vi "MGCC_Resync_main.vi"() -> ()   [LabVIEW 2016]
doc: "-----------------------------------------------------------------------------------------------------------------------\nCopyright <2019> <The University of Tennessee at Knoxville and the University of Tennessee Research Foundation>\nThis software is released under BSD-3 \nhttps://opensource.org/licenses/BSD-3-Clause \nAdditional license options available at https://utrf.tennessee.edu/industry/sample-agreements/\n-----------------------------------------------------------------------------------------------------------------------\n\nSimplified version of resynchronization, without support on dynamic boundary"
uses:
  Finite State Machine/Sub-VIs/MGCC_FntStaMach_gobal.vi
  <vilib>/Utility/error.llb/Error Cluster From Error Code.vi
  Communication/Global communication output.vi
  MGCC_Resync_global.vi
  Communication/Global communication.vi
  <vilib>/ErrorRing/Error Ring.xnode
panel:
  out "Resync Iterations":i16
  out "Critical_switch_first":i16
  out "resync_switch":i32[](array[numeric])
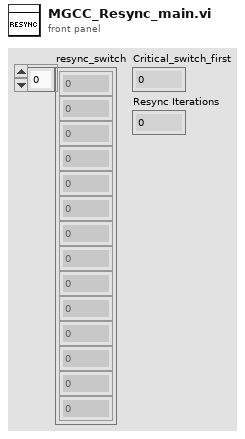
[diagram p1: front panel]
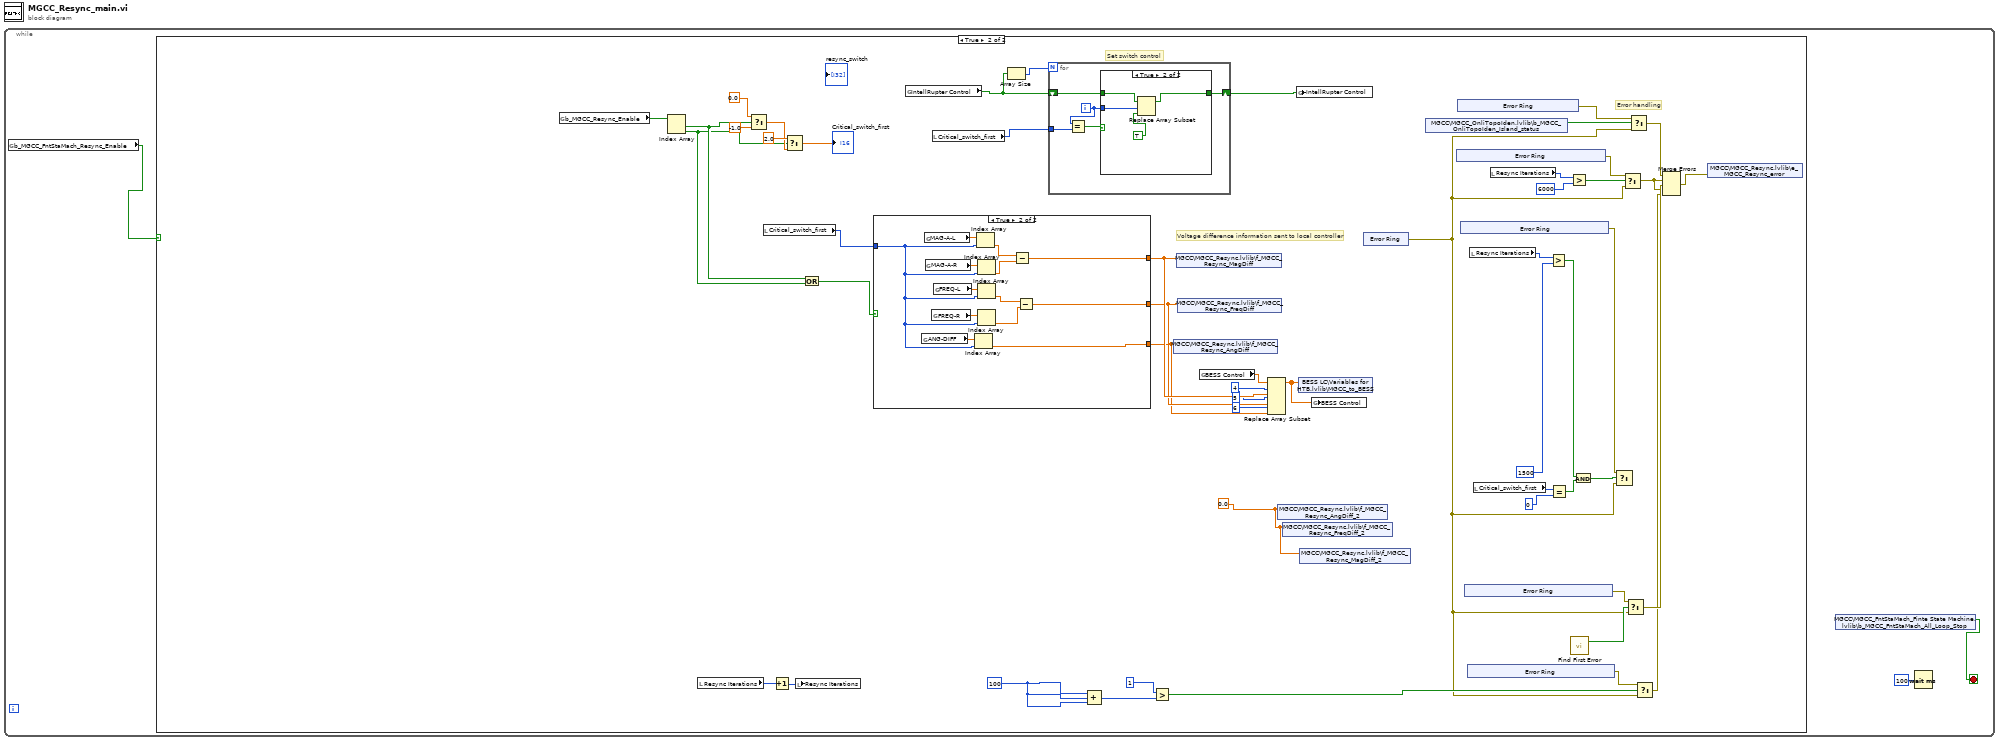
[diagram p0: block diagram]
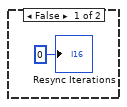
[diagram p2: hidden frame]
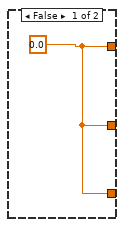
[diagram p3: hidden frame]
diagram:
  n1 = while {
    stop <- w2 stop-if-true
    n2 = global read "MGCC_FntStaMach_gobal.vi" "b_MGCC_FntStaMach_Resync_Enable"() -> (w1:bool)
    n3 = case shown="True" w1 {
      frame False {
        "Resync Iterations" <- i16 0 ("Resync Iterations")
      }
      frame True {
        w35 = 100 ("y")
        w28 = 0.0
        # "Set switch control"
        # "Error handling"
        # "Voltage difference information sent to local controller"
        n4 = global read "MGCC_Resync_global.vi" "b_MGCC_Resync_Enable"() -> (w18:bool[])
        n5 = Index Array(array=w18) -> (element #1=w9:bool, element #2=w8:bool)  [unwired: 2 in]
        n6 = local read "Resync Iterations"() -> (w56:i16)
        n7 = Select(t=0.0 ("f"), s=w9, f=-1.0) -> (s? t:f=w15:dbl)
        n8 = local read "Critical_switch_first"() -> (w12:i16)
        n9 = Increment(x=w56) -> (x+1=w55:i16)
        n10 = Select(t=2.0 ("f"), s=w8, f=w15) -> (s? t:f=→"Critical_switch_first":dbl)
        n11 = local write "Resync Iterations"(w55) -> ()
        n12 = Or(x=w9, y=w8) -> (x .or. y?=w10:bool)
        n13 = case shown="True" w10 {
          tunnel: [w57 w61] -> w23
          tunnel: [w57 w60] -> w22
          tunnel: [w57 w59] -> w21
          tunnel: w12 -> [_ w58]
          frame False {
            w57 = 0.0
          }
          frame True {
            n14 = global read "Global communication.vi" "ANG-DIFF"() -> (w66:dbl[])
            n15 = global read "Global communication.vi" "MAG-A-L"() -> (w70:dbl[])
            n16 = global read "Global communication.vi" "MAG-A-R"() -> (w69:dbl[])
            n17 = global read "Global communication.vi" "FREQ-R"() -> (w67:dbl[])
            n18 = global read "Global communication.vi" "FREQ-L"() -> (w68:dbl[])
            n19 = Index Array(array=w66, index=w58) -> (element=w59:dbl)
            n20 = Index Array(array=w70, index=w58) -> (element=w65:dbl)
            n21 = Index Array(array=w69, index=w58) -> (element=w64:dbl)
            n22 = Index Array(array=w67, index=w58) -> (element=w62:dbl)
            n23 = Index Array(array=w68, index=w58) -> (element=w63:dbl)
            n24 = Subtract(x=w65, y=w64) -> (x-y=w61:dbl)
            n25 = Subtract(x=w63, y=w62) -> (x-y=w60:dbl)
          }
        }
        n26 = global read "Global communication output.vi" "IntellRupter Control"() -> (w6:bool[])
        n27 = local read "Critical_switch_first"() -> (w11:i16)
        n28 = Array Size(array=w6) -> (size(s)=w7:i32)
        n29 = for {
          N: w7 -> [_]
          shift-right: [w73] -> w27
          shift-left: w6 -> [w74]
          tunnel: w11 -> [w72]
          i -> [w71]
          n30 = Equal?(x=w71, y=w72) -> (x = y?=w75:bool)
          n31 = case shown="True" w75 {
            tunnel: w74 -> [w76 w80]
            tunnel: w71 -> [_ w79]
            tunnel: [w76 w78] -> w73
            frame False {
            }
            frame True {
              n32 = Replace Array Subset(array=w80, new element=TRUE ("new element/subarray"), index=w79) -> (w78:bool[])
            }
          }
        }
        n33 = Compound Arithmetic op=unknown(w35, w35, w35) -> (w34:i32)
        n34 = Greater?(x=1 ("y"), y=w34) -> (0:w32:bool)
        n35 = shared-variable "MGCC\\MGCC_Resync.lvlib\\f_MGCC_Resync_AngDiff"(w21) -> ()  [unwired: 1 in, 1 out]
        n36 = shared-variable "MGCC\\MGCC_Resync.lvlib\\f_MGCC_Resync_MagDiff"(w23) -> ()  [unwired: 1 in, 1 out]
        n37 = shared-variable "MGCC\\MGCC_Resync.lvlib\\f_MGCC_Resync_FreqDiff"(w22) -> ()  [unwired: 1 in, 1 out]
        n38 = global read "Global communication output.vi" "BESS Control"() -> (w24:dbl[])
        n39 = Replace Array Subset(array=w24, new element #1=w23, index #1=4 ("index"), new element #2=w22, index #2=5 ("index"), new element #3=w21, index #3=6 ("index")) -> (w25:dbl[])
        n40 = shared-variable "MGCC\\MGCC_Resync.lvlib\\f_MGCC_Resync_AngDiff_2"(w28) -> ()  [unwired: 1 in, 1 out]
        n41 = shared-variable "MGCC\\MGCC_Resync.lvlib\\f_MGCC_Resync_FreqDiff_2"(w28) -> ()  [unwired: 1 in, 1 out]
        n42 = global write "Global communication output.vi" "IntellRupter Control"(w27) -> ()
        n43 = shared-variable "BESS LC\\Variables for HTB.lvlib\\MGCC_to_BESS"(w25) -> ()  [unwired: 1 in, 1 out]
        n44 = shared-variable "MGCC\\MGCC_Resync.lvlib\\f_MGCC_Resync_MagDiff_2"(w28) -> ()  [unwired: 1 in, 1 out]
        n45 = global write "Global communication output.vi" "BESS Control"(w25) -> ()
        n46 = xnode "Error Ring"() -> ("error out"=w30:errorcluster)
        n47 = shared-variable "MGCC\\MGCC_OnliTopoIden.lvlib\\b_MGCC_OnliTopoIden_Island_status"() -> (w50:bool)  [unwired: 1 in, 1 out]
        n48 = xnode "Error Ring"() -> ("error out"=w51:errorcluster)
        n49 = xnode "Error Ring"() -> ("error out"=w49:errorcluster)
        n50 = xnode "Error Ring"() -> ("error out"=w36:errorcluster)
        n51 = xnode "Error Ring"() -> ("error out"=w47:errorcluster)
        n52 = xnode "Error Ring"() -> ("error out"=w31:errorcluster)
        n53 = local read "Resync Iterations"() -> (w42:i16)
        n54 = local read "Critical_switch_first"() -> (w41:i16)
        n55 = local read "Resync Iterations"() -> (w54:i16)
        n56 = Greater?(x=w42, y=i16 1500) -> (0:w39:bool)
        n57 = Equal?(x=w41, y=i16 0) -> (x = y?=w38:bool)
        n58 = Greater?(x=w54, y=i16 6000) -> (0:w52:bool)
        n59 = call <vilib>:"Find First Error.vi"() -> ("error?"=w48:bool)  [unwired: 4 in, 1 out]
        n60 = And(x=w39, y=w38) -> (x .and. y?=w37:bool)
        n61 = Select(t=w36, s=w37, f=w30) -> ()  [unwired: 1 out]
        n62 = Select(t=w51, s=w52, f=w30) -> (s? t:f=w5:errorcluster)
        n63 = Select(t=w47, s=w48, f=w30) -> (s? t:f=w45:errorcluster)
        n64 = Select(t=w49, s=w50, f=w30) -> (s? t:f=w46:errorcluster)
        n65 = Select(t=w31, s=w32, f=w30) -> (s? t:f=w29:errorcluster)
        n66 = Merge Errors(w46, w5, w45, w5, w29) -> (w44:errorcluster)
        n67 = shared-variable "MGCC\\MGCC_Resync.lvlib\\e_MGCC_Resync_error"(error in=w44) -> ()  [unwired: 2 out]
      }
    }
    n68 = shared-variable "MGCC\\MGCC_FntStaMach_Finte State Machine.lvlib\\b_MGCC_FntStaMach_All_Loop_Stop"() -> (w2:bool)  [unwired: 1 in, 1 out]
    n69 = Wait (ms)(milliseconds to wait=u32 100) -> ()  [unwired: 1 out]
  }
